vi "TestPurePursuit.vi"() -> ()   [LabVIEW 2017]
uses:
  Shared/RobotNeededPathData.ctl
panel:
  in  "SlowSpeed":dbl=15.0
  in  "SlowDistanceAtEnd":dbl=12.0
  in  "Speed/Curve":dbl=2.5 format="%#_13g"
  in  "Start Location":cluster{dbl, dbl}
  in  "Backwards":bool
  out "Left/Right Power":cluster{"LeftValue":dbl, "RightValue":dbl}(graph)={"LeftValue"=0.39187271772375715, "RightValue"=0.3900748910335044}
  out "Target Vel":dbl(graph)=36.480000000000004
  in  "Gains":T1={"FFV"=0.0055, "FFA"=0.0025, "Vel PID"={"P"=0.005, "I"=0.0, "D"=0.0}} {"Vel PID"."D" format="%.5f"; "Vel PID"."I" format="%.3f"; "Vel PID"."P" format="%.3f"}
  out "Graph":cluster{cluster{"x":dbl, "y":dbl}[]}[](graph)=[{[{"x"=0.0, "y"=0.0}, {"x"=5.991608726623139, "y"=-0.005878191574676967}, {"x"=11.98111729667086, "y"=-0.01322303172743175}, {"x"=17.9659259206227, "y"=-0.02385999015293685}, {"x"=23.942248410915674, "y"=-0.040439667526228545}, {"x"=29.904157994783606, "y"=-0.06711040792813325}, {"x"=35.84211414292494, "y"=-0.11055780275487107}, {"x"=41.740585165239246, "y"=-0.18165209285327164}, {"x"=47.574194042361334, "y"=-0.2981916290303774}, {"x"=53.30130982399895, "y"=-0.48928276276907645}, {"x"=58.85377122969291, "y"=-0.8027111915740697}, {"x"=64.11964097247744, "y"=-1.3168296991668145}, {"x"=68.91541648341607, "y"=-2.160145654783597}, {"x"=72.9400613729898, "y"=-3.5434949475732958}, {"x"=75.69971482115338, "y"=-5.812723483703834}, {"x"=77.38429771853998, "y"=-9.535134937889756}, {"x"=78.4149497646454, "y"=-14.14131666738604}, {"x"=79.04935476791528, "y"=-19.282833668630552}, {"x"=79.44610301858104, "y"=-24.745051434766317}, {"x"=79.70436521224107, "y"=-30.393538121495602}, {"x"=79.88871692993212, "y"=-36.140413741315704}, {"x"=80.04525642106013, "y"=-41.92238544113582}, {"x"=80.21311376487884, "y"=-47.68494831631544}, {"x"=80.43424752461144, "y"=-53.368750639803565}, {"x"=80.76394291300683, "y"=-58.89474290734003}, {"x"=81.28462688797174, "y"=-64.14441887049676}, {"x"=82.12646959763643, "y"=-68.93019649615196}, {"x"=83.49992920548148, "y"=-72.94852260956638}, {"x"=85.74837002989447, "y"=-75.70398064383866}, {"x"=89.4339035584217, "y"=-77.38543491294872}, {"x"=93.97791377751095, "y"=-78.4132479398045}, {"x"=99.01640277139329, "y"=-79.04437298904456}, {"x"=104.30899121309002, "y"=-79.43659123045325}, {"x"=109.67882618697212, "y"=-79.68795831668827}, {"x"=114.968367130826, "y"=-79.86131486176646}, {"x"=120.0, "y"=-80.0}]}, {[{"x"=7.718790114245136, "y"=-0.005088272808129804}, {"x"=19.71878238471526, "y"=-0.01870842909386336}]}, {[{"x"=20.965914376183157, "y"=-0.03218264021032251}]}, {[{"x"=20.718790114245138, "y"=-0.005088272808129804}, {"x"=18.236011041119454, "y"=7.636120006994021}, {"x"=11.736011041119454, "y"=12.358646439028865}, {"x"=3.701569187370821, "y"=12.358646439028867}, {"x"=-2.7984308126291797, "y"=7.636120006994022}, {"x"=-5.281209885754864, "y"=-0.005088272808128212}, {"x"=-2.7984308126291815, "y"=-7.646296552610279}, {"x"=3.7015691873708176, "y"=-12.368822984645126}, {"x"=11.73601104111945, "y"=-12.368822984645128}, {"x"=18.236011041119454, "y"=-7.646296552610283}, {"x"=20.718790114245138, "y"=-0.005088272808132988}]}, {[{"x"=7007.15916945149, "y"=-7007.3944372521}, {"x"=5668.866027967043, "y"=-2888.5516677908654}, {"x"=2165.169096649888, "y"=-342.9668419470745}, {"x"=-2165.638483015526, "y"=-342.9668419470736}, {"x"=-5669.33541433268, "y"=-2888.5516677908645}, {"x"=-7007.628555817128, "y"=-7007.394437252099}, {"x"=-5669.3354143326815, "y"=-11126.237206713335}, {"x"=-2165.6384830155275, "y"=-13671.822032557126}, {"x"=2165.169096649887, "y"=-13671.822032557127}, {"x"=5668.866027967042, "y"=-11126.237206713336}, {"x"=7007.15916945149, "y"=-7007.394437252102}]}]
  in  "Max Accel":dbl=60.0 format="%#_13g"
  in  "MaxVel":dbl(slide)=104.8951048951049 scale=0.0..150.0
  in  "LookAhead":dbl=13.0
  in  "Path":cluster{"x":dbl, "y":dbl}[](array[cluster])=[{"x"=0.0, "y"=0.0}, {"x"=80.0, "y"=0.0}, {"x"=80.0, "y"=-80.0}, {"x"=120.0, "y"=-80.0}]
  in  "Config":T2={"Gear Reduction"=8.7, "Wheel Radius (m)"=0.076, "# Motors"=3, "coeff of friction"=0.1, "Mass (kg)"=55.0, "Motor"={"Ke (V)"=0.0183, "R (ohms)"=0.14, "KT (Nm/A)"=0.0183, "Tf (Nm)"=0.015}}
  # ".007"
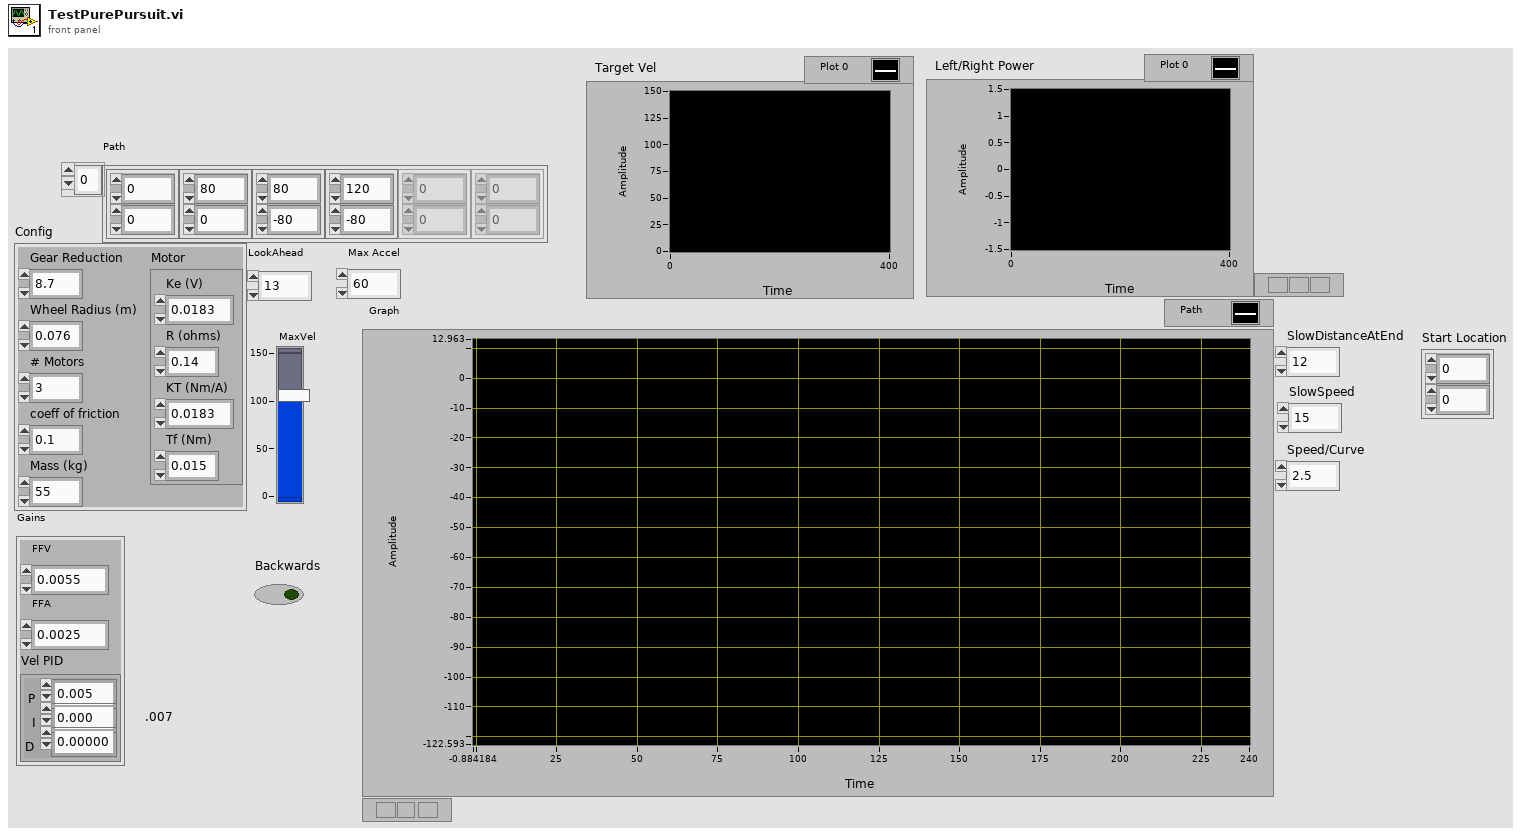
[diagram p1: front panel]
types:
  T1 = cluster{"FFV":dbl, "FFA":dbl, "Vel PID":cluster{"P":dbl, "I":dbl, "D":dbl}}
  T2 = cluster{"Gear Reduction":dbl, "Wheel Radius (m)":dbl, "# Motors":u32, "coeff of friction":dbl, "Mass (kg)":dbl, "Motor":cluster{"Ke (V)":dbl, "R (ohms)":dbl, "KT (Nm/A)":dbl, "Tf (Nm)":dbl}}
  T3 = typedef "RobotNeededPathData.ctl" = cluster{"Path":cluster{dbl, dbl}[], "MaxVel":dbl, "MaxAccel":dbl, "Backwards?":bool, "PointSpacing":dbl, "LookaheadDist":dbl, "Speed/Curve":dbl, "SlowDistanceAtEnd":dbl, "SlowSpeed":dbl}
  T4 = cluster{"Left Distance":dbl, "Right Distance":dbl, "dx/dt":dbl, "dx/dt":dbl, dbl, "Location":cluster{dbl, dbl}}
  T5 = cluster{"Left Distance":dbl, "Right Distance":dbl, "dx/dt":dbl, "dx/dt":dbl, dbl, cluster{dbl, dbl}}
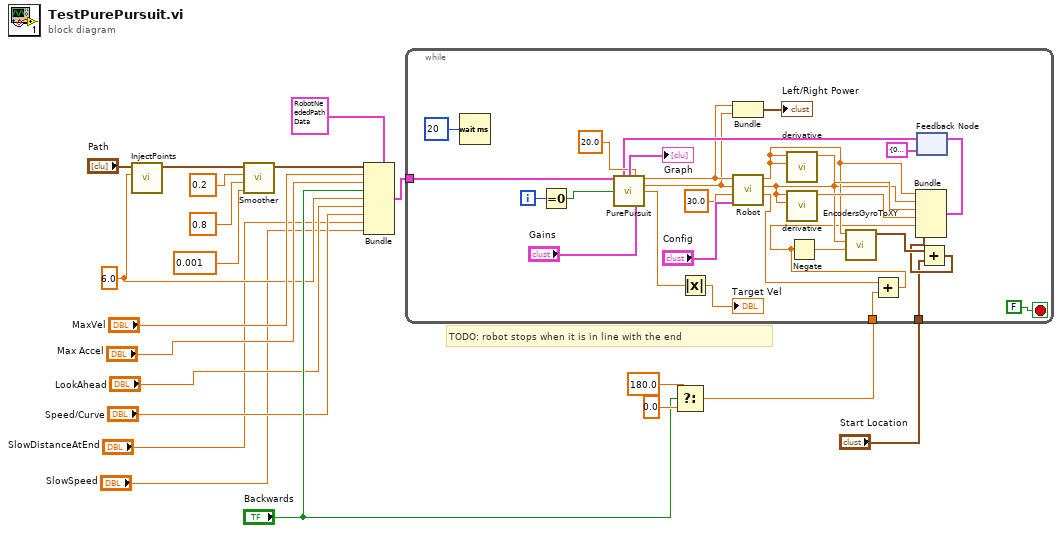
[diagram p0: block diagram]
diagram:
  w5 = 6.0 ("Distance")
  # "TODO: robot stops when it is in line with the end"
  n1 = call "InjectPoints.vi"("Spacing"=w5, "Path"="Path") -> ("Path out"=w15:cluster{dbl, dbl}[])  [unwired: 9 in]
  n2 = call "Smoother.vi"("tolerance"=0.001, "B"=0.8, "A"=0.2, "Path"=w15) -> ("SmoothPath"=w14:cluster{dbl, dbl}[])  [unwired: 7 in]
  n3 = Bundle(cluster=T3 {"Path"=[], "MaxVel"=0.0, "MaxAccel"=0.0, "Backwards?"=FALSE, "PointSpacing"=0.0, "LookaheadDist"=0.0, "Speed/Curve"=1.8, "SlowDistanceAtEnd"=12.0, "SlowSpeed"=15.0} ("RobotNeededPathData"), "Path"=w14, "MaxVel"="MaxVel", "MaxAccel"="Max Accel", "Backwards?"="Backwards", "PointSpacing"=w5, "LookaheadDist"="LookAhead", "Speed/Curve"="Speed/Curve", "SlowDistanceAtEnd"="SlowDistanceAtEnd", "SlowSpeed"="SlowSpeed") -> (w16:T3)
  n4 = Select(t=180.0, s="Backwards", f=0.0) -> (s? t:f=w11:dbl)
  n5 = while {
    tunnel: w16 -> [w23]
    tunnel: w11 -> [w29]
    tunnel: "Start Location" -> [w24]
    i -> [w35]
    stop <- FALSE stop-if-true
    n6 = Wait (ms)(milliseconds to wait=u32 20) -> ()  [unwired: 1 out]
    n7 = Equal To 0?(x=w35) -> (x = 0?=w34:bool)
    n8 = feedback #1(T4 {"Left Distance"=0.0, "Right Distance"=0.0, "dx/dt"=0.0, "dx/dt"=0.0, 0.0, "Location"={0.0, 0.0}}) -> (w37:T4)
    n9 = call "PurePursuit.vi"("RobotNeededPathData"=w23, "SensorData"=w37, "Trackwidth"=20.0, "Reset"=w34, "Gains"="Gains") -> ("Graph"=→"Graph":cluster{cluster{"x":dbl, "y":dbl}[]}[], "LeftValue"=w33:dbl, "RightValue"=w32:dbl, "TargetVel"=w22:dbl)  [unwired: 6 in, 1 out]
    n10 = Absolute Value(x=w22) -> (abs(x)=→"Target Vel":dbl)
    n11 = Bundle("LeftValue"=w33, "RightValue"=w32) -> (→"Left/Right Power":cluster{"LeftValue":dbl, "RightValue":dbl})  [unwired: 1 in]
    n12 = call "Robot.vi"("Config"="Config", "WheelBase"=30.0, "Right Value"=w32, "Left Value"=w33) -> ("Angle"=w30:dbl, "Right Distance"=w36:dbl, "Left Distance"=w39:dbl)  [unwired: 5 in]
    n13 = call "derivative.vi"("Starting value"=w39, "x"=w39) -> ("dx/dt"=w41:dbl)  [unwired: 9 in]
    n14 = call "derivative.vi"("Starting value"=w36, "x"=w36) -> ("dx/dt"=w40:dbl)  [unwired: 9 in]
    n15 = Add(x=w30, y=w29) -> (x+y=w28:dbl)
    n16 = Negate(x=w28) -> (-x=w38:dbl)
    n17 = call "EncodersGyroToXY.vi"("Angle (degrees)"=w38, "Right Distance"=w36, "Left Distance"=w39) -> ("Location"=w26:cluster{dbl, dbl})  [unwired: 8 in]
    n18 = Add(x=w26, y=w24) -> (x+y=w25:cluster{dbl, dbl})
    n19 = Bundle("Left Distance"=w39, "Right Distance"=w36, "dx/dt"=w41, "dx/dt"=w40, w28, w25) -> (w46:T5)  [unwired: 1 in]
    n20 = feedback-in #1(w46) -> ()
  }
